vi "Create Pattern Script - WR Frame.vi"(8 "error in (no error)":errorcluster, 10 "FRM Data":T1 {"Addr" format="%x"; "Data" format="%x"}, 11 "SPI 4W Pattern Creator in":refnum<class "SPI 4W Pattern Creator.lvclass">) -> (0 "error out":errorcluster, 2 "String":string, 3 "SPI 4W Pattern Creator out":refnum<class "SPI 4W Pattern Creator.lvclass">)   [LabVIEW 2018, in "SPI 4W Pattern Creator.lvlib" / "SPI 4W Pattern Creator.lvclass"]
uses:
  SPI 4W Pattern Creator.lvclass
  Ctls/Frame Data - SPI_3W.ctl
  Ctls/RW Options.ctl
  Protocols/SPI Root Pattern Creator.lvlibp/Plugins/SouceCode/SPI_Pattern Creator/SPI Root/Special Frame Type.ctl
  Protocols/SPI Root Pattern Creator.lvlibp/Plugins/SouceCode/SPI_Pattern Creator/SPI Root/SPI Root Pattern Creator.lvclass
  C:/P4 Workspace/PC Client/Solutions/5g_eap/trunk/1.0/HiSi5GmmWave/Pattern_Gen_Tool/Plugins/Protocols/SPI Root Pattern Creator.lvlibp/Plugins/SouceCode/SPI_Pattern Creator/SPI Root/SPI Root Pattern Creator.lvclass
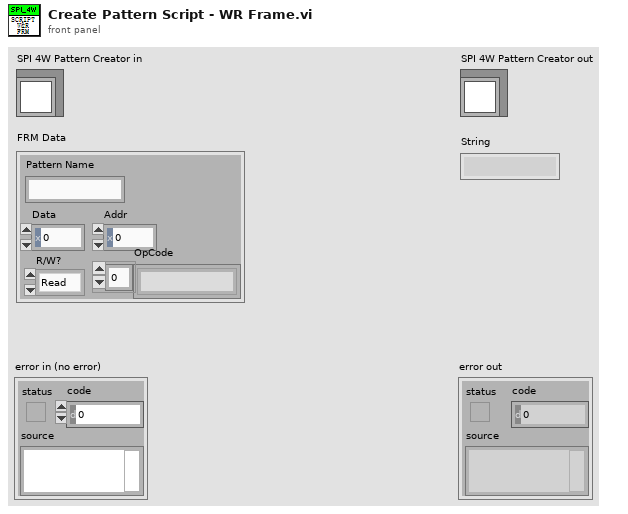
[diagram p1: front panel]
types:
  T1 = typedef "Frame Data - SPI_3W.ctl" = cluster{"Pattern Name":string, "Data":u16, "Addr":u16, "OpCode":string[], "R/W?":T2}
  T2 = typedef "RW Options.ctl" = enum16{"Read", "Write", "R/W"}
  T3 = typedef "SPI Root Pattern Creator.lvlibp/SPI Root Pattern Creator.lvclass/Special Frame Type.ctl" = enum16{"SPI 4W FRM Start", "SPI 4W Wait", "SPI 4W FRM End", "SPI 4W Write Cmd", "SPI Rd Collect Cmd", "SPI Rd Value Cmd", "SPI 3W FRM Start", "SPI 3W Write Cmd", "SPI 3W FRM End", "SPI 3W Wait", "SPI 3W Rd Cmd"}
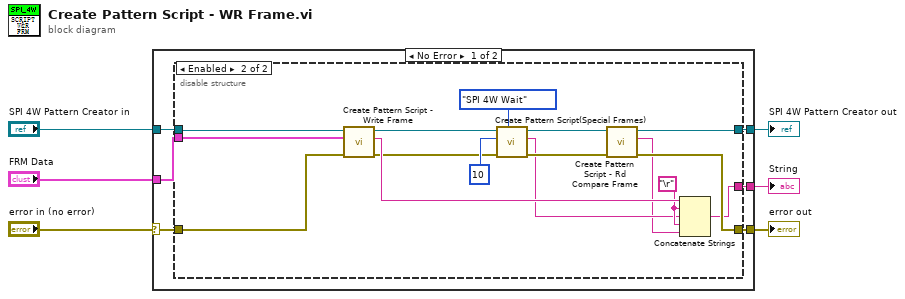
[diagram p0: block diagram]
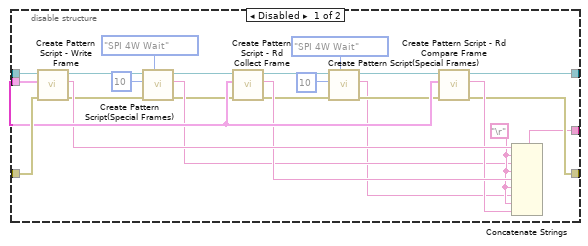
[diagram p2: hidden frame]
diagram:
  n1 = case shown="No Error" "error in (no error)" {
    selector: "error in (no error)" -> [w11 w53]
    tunnel: "SPI 4W Pattern Creator in" -> [w12 w54]
    tunnel: "FRM Data" -> [w10 _]
    tunnel: [w9 w54] -> w3
    tunnel: [w8 w53] -> w2
    tunnel: [w7 _] -> w1
    frame No Error {
      n2 = disable-structure shown="Enabled" {
        disable-tunnel: w12 -> [w36 w44]
        disable-tunnel: w11 -> [w35 w46]
        disable-tunnel: w10 -> [w34 w45]
        disable-tunnel: [w29 w41] -> w9
        disable-tunnel: [w28 w40] -> w8
        disable-tunnel: [w27 w37] -> w7
        frame Disabled {
          w30 = "\r"
          n3 = call-dynamic "Create Pattern Script - Write Frame.vi"("error in (no error)"=w35, "FRM Data"=w34, "SPI 4W Pattern Creator in"=w36) -> ("error out"=w22:errorcluster, "String"=w33:string, "SPI 4W Pattern Creator out"=w26:refnum<class "SPI 4W Pattern Creator.lvclass">)  [unwired: 6 in]
          n4 = call "Create Pattern Script(Special Frames).vi"("Special Frame Type"=Special_Frame_Type."SPI 4W Wait", "error in (no error)"=w22, "Num of Timeset"=u32 10, "SPI Root Pattern Creator in"=w26) -> ("error out"=w23:errorcluster, "String out"=w24:string, "SPI Root Pattern Creator out"=w25:refnum<class "SPI 4W Pattern Creator.lvclass">)  [unwired: 5 in]
          n5 = call-dynamic "Create Pattern Script - Rd Collect Frame.vi"("error in (no error)"=w23, "FRM Data"=w34, "SPI 4W Pattern Creator in"=w25) -> ("error out"=w17:errorcluster, "String"=w32:string, "SPI 4W Pattern Creator out"=w16:refnum<class "SPI 4W Pattern Creator.lvclass">)  [unwired: 6 in]
          n6 = call "Create Pattern Script(Special Frames).vi"("Special Frame Type"=Special_Frame_Type."SPI 4W Wait", "error in (no error)"=w17, "Num of Timeset"=u32 10, "SPI Root Pattern Creator in"=w16) -> ("error out"=w18:errorcluster, "String out"=w15:string, "SPI Root Pattern Creator out"=w19:refnum<class "SPI 4W Pattern Creator.lvclass">)  [unwired: 5 in]
          n7 = call-dynamic "Create Pattern Script - Rd Compare Frame.vi"("error in (no error)"=w18, "FRM Data"=w34, "SPI 4W Pattern Creator in"=w19) -> ("error out"=w28:errorcluster, "String"=w31:string, "SPI 4W Pattern Creator out"=w29:refnum<class "SPI 4W Pattern Creator.lvclass">)  [unwired: 6 in]
          n8 = Concatenate Strings(w33, w30, w24, w30, w32, w30, w15, w30, w31) -> (w27:string)
        }
        frame Enabled {
          w51 = "\r"
          n9 = call-dynamic "Create Pattern Script - Write Frame.vi"("error in (no error)"=w46, "FRM Data"=w45, "SPI 4W Pattern Creator in"=w44) -> ("error out"=w43:errorcluster, "String"=w52:string, "SPI 4W Pattern Creator out"=w42:refnum<class "SPI 4W Pattern Creator.lvclass">)  [unwired: 6 in]
          n10 = call "Create Pattern Script(Special Frames).vi"("Special Frame Type"=Special_Frame_Type."SPI 4W Wait", "error in (no error)"=w43, "Num of Timeset"=u32 10, "SPI Root Pattern Creator in"=w42) -> ("error out"=w48:errorcluster, "String out"=w39:string, "SPI Root Pattern Creator out"=w49:refnum<class "SPI 4W Pattern Creator.lvclass">)  [unwired: 5 in]
          n11 = call-dynamic "Create Pattern Script - Rd Compare Frame.vi"("error in (no error)"=w48, "SPI 4W Pattern Creator in"=w49) -> ("error out"=w40:errorcluster, "String"=w38:string, "SPI 4W Pattern Creator out"=w41:refnum<class "SPI 4W Pattern Creator.lvclass">)  [unwired: 7 in]
          n12 = Concatenate Strings(w52, w51, w39, w51, w38) -> (w37:string)
        }
      }
    }
    frame Error {
    }
  }
  "error out" <- w2
  "SPI 4W Pattern Creator out" <- w3
  "String" <- w1
